vi "Update VI Properties.vi"() -> ()   [LabVIEW 2016, in "update vi properties.lvlib"]
uses:
  update vi properties.lvlib
  _support/user action.ctl
  _support/Event Data.ctl
  _support/Cluster_Data.ctl
  <vilib>/picture/picture.llb/imagedata.ctl
panel:
  in  "Add copyright":bool
  out "Inline?":bool
  out "Reentrant?":bool
  in  "Abbr. if class in lib":bool=TRUE
  in  "Adjust all Controls & Indicators":bool=TRUE
  in  "Prompt?":bool
  in  "Set all VIs":bool
  in  "Load":bool
  in  "Error in":errorcluster
  in  "Event Data":T1={"Action"=enum."Apply", "VI Index"=0}
  in  "Controls":string[][](table)
  in  "Indicators":string[][](table)
  in  "Help Tag":string
  in  "Help Path":string
  out "Path to VI":string
  in  "VI Description":string
  out "VI Conn Pane":picture
  in  "Listbox with VIs":i32(listbox)=-1 caption="Select a VI to View/Edit Properties:"
  in  "Action":T2=enum."Apply"
  in  "OK":bool
  in  "Cancel":bool
  in  "Apply":bool
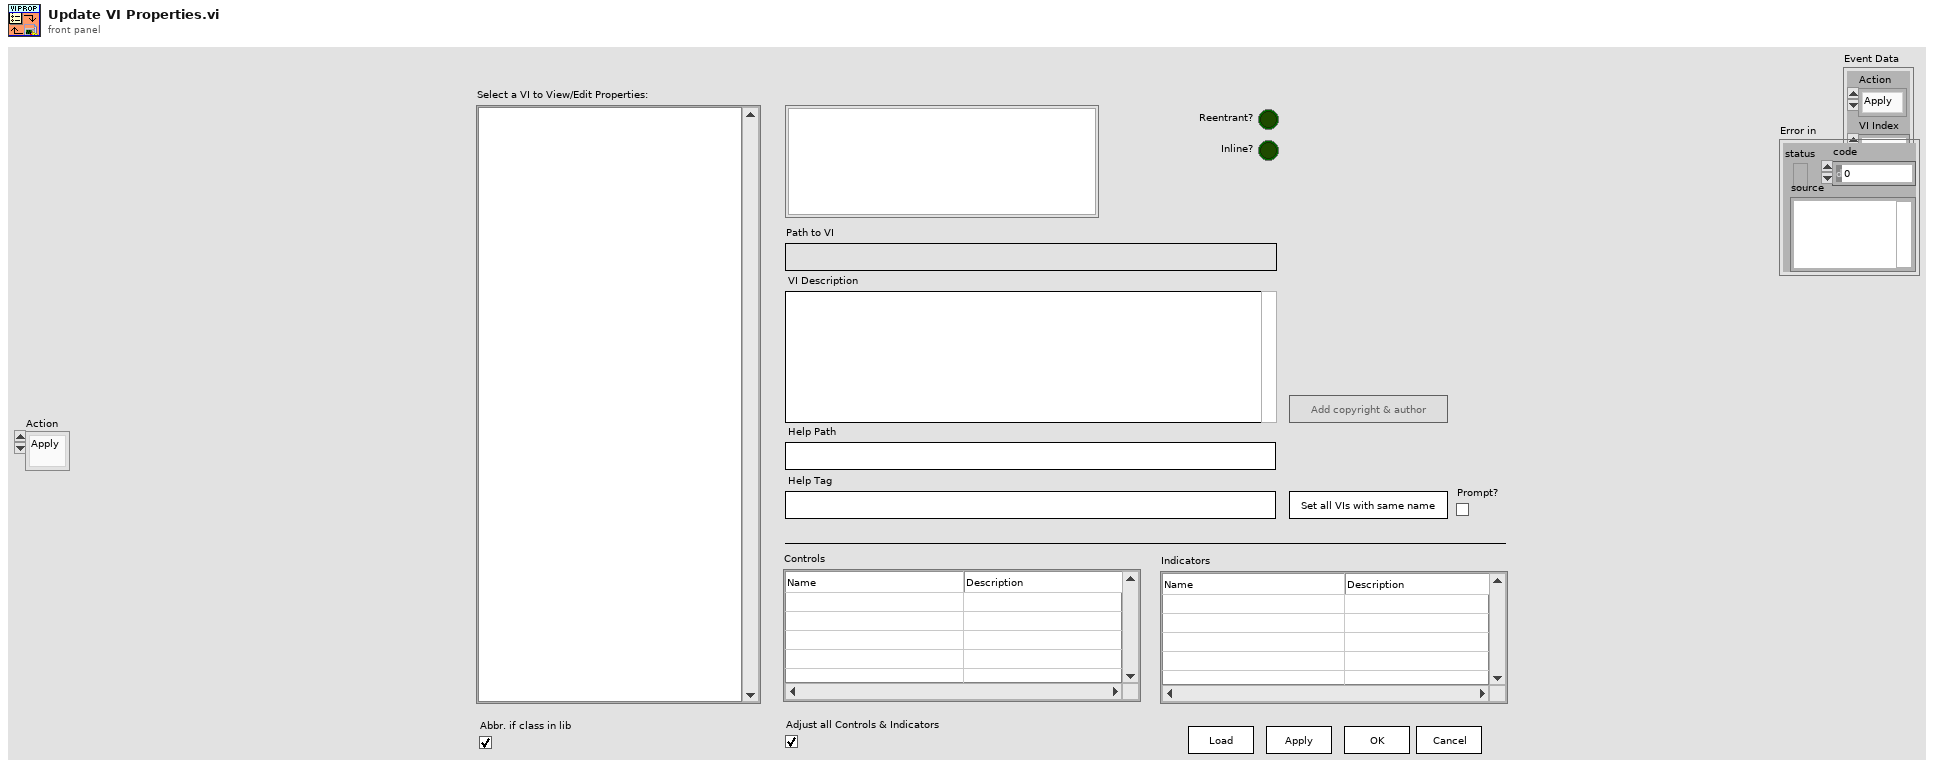
[diagram p1: front panel]
types:
  T1 = typedef "update vi properties.lvlib/Event Data.ctl" = cluster{"Action":T2, "VI Index":i32}
  T2 = typedef "update vi properties.lvlib/user action.ctl" = enum16{"Load VIs", "VI Selected", "Value Changed", "Set all VIs", "Controls/Indicator Changed", "Open VI", "Apply", "Cancel"}
  T3 = typedef "update vi properties.lvlib/Cluster_Data.ctl" = cluster{"changed?":bool, "VI Data":string[], "Controls":string[][], "Indicator":string[][], "Conpane Img":T4}
  T4 = typedef "imagedata.ctl" = cluster{"image type":i32, "image depth":i32, "image":u8[], "mask":u8[], "colors":u32[], "Rectangle":cluster{"left":i16, "top":i16, "right":i16, "bottom":i16}}
  T5 = enum32{"invalid VI type", "Standard VI", "Control VI", "Global VI", "Polymorphic VI", "Configuration VI", "SubSystem", "Facade VI", "Method VI", "Statechart Diagram VI"}
  T6 = enum8{"Enabled", "Disabled", "Disabled and Grayed Out"}
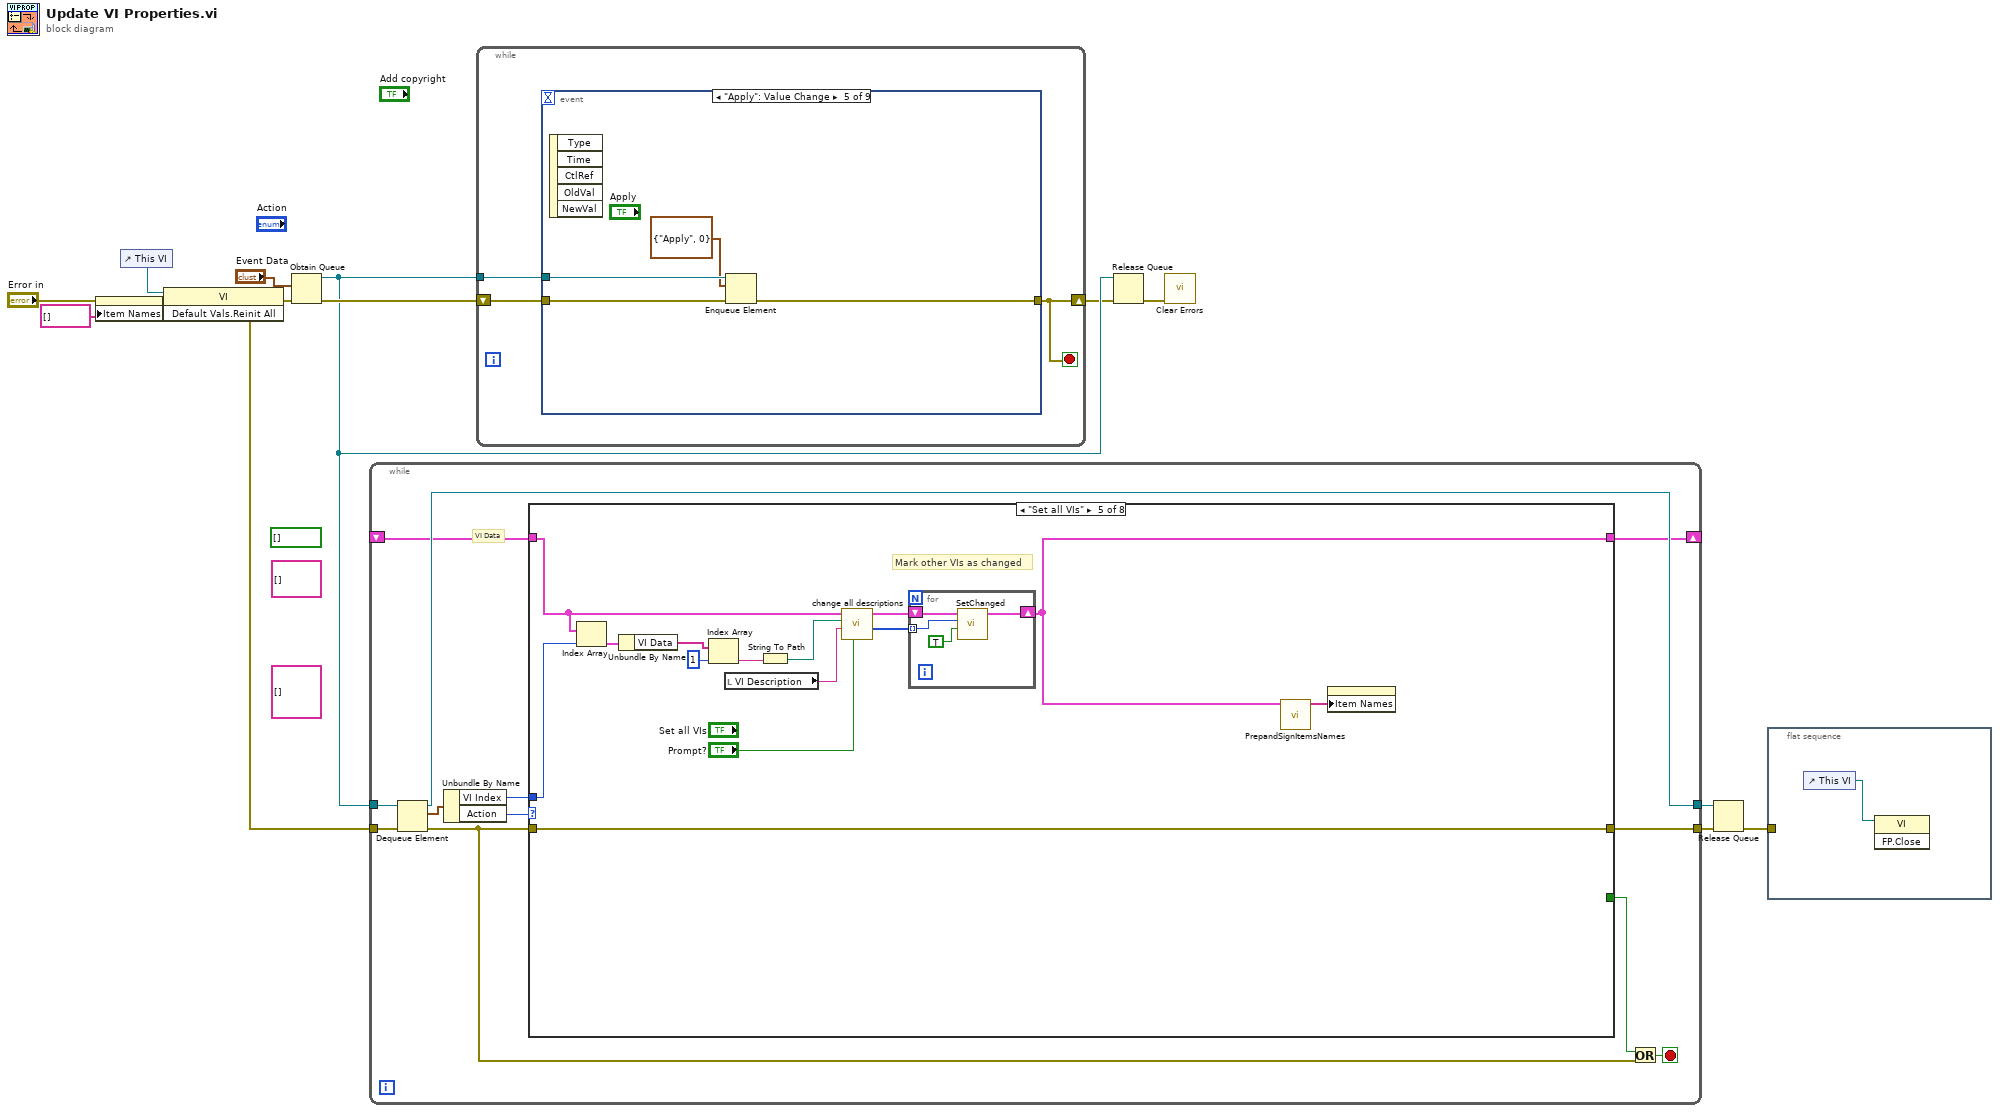
[diagram p0: block diagram]
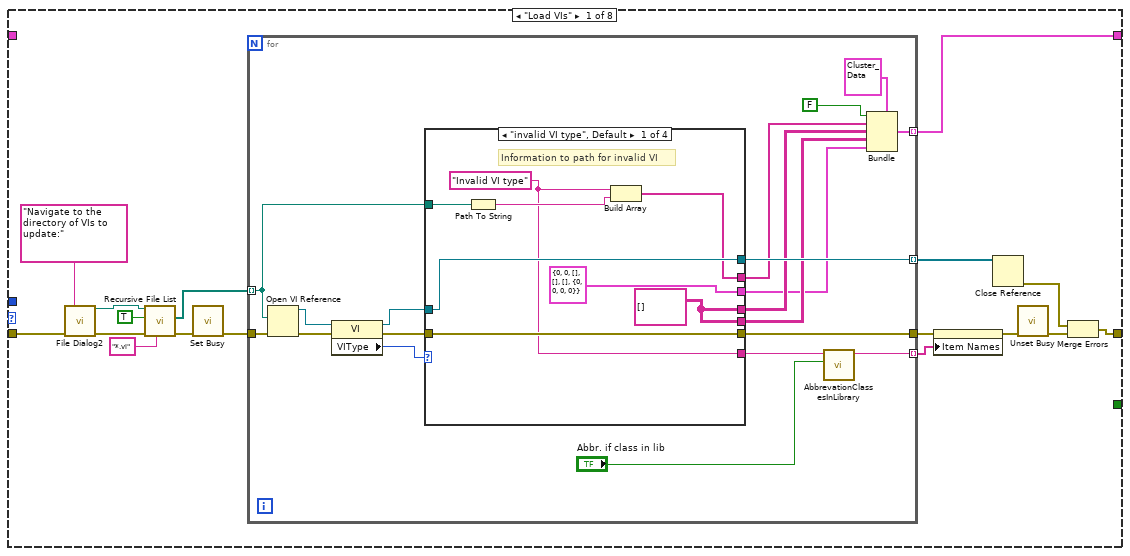
[diagram p2: hidden frame]
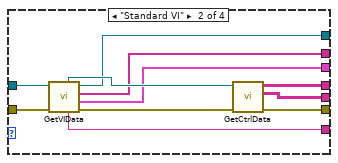
[diagram p3: hidden frame]
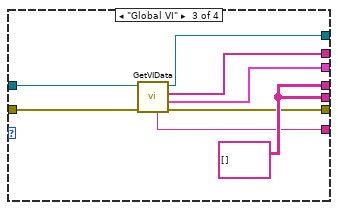
[diagram p4: hidden frame]
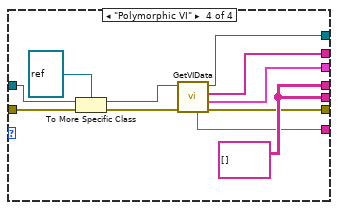
[diagram p5: hidden frame]
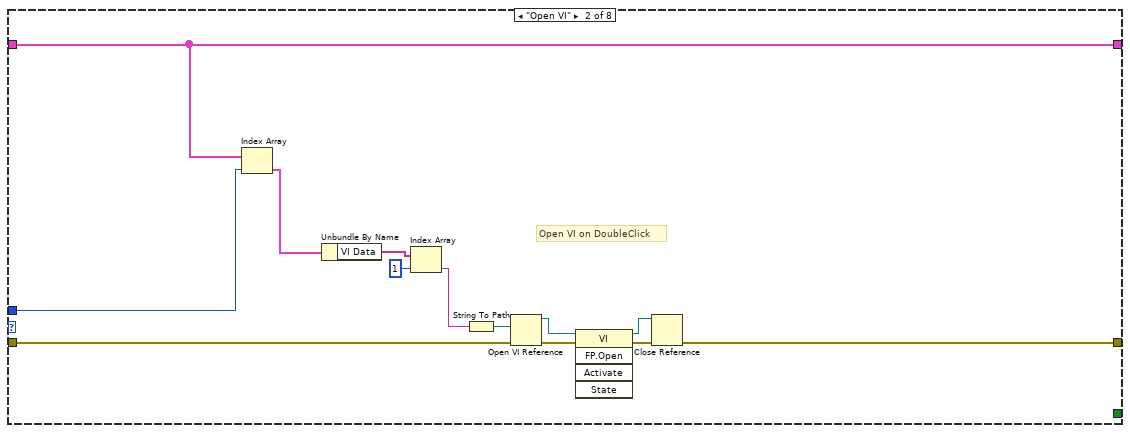
[diagram p6: hidden frame]
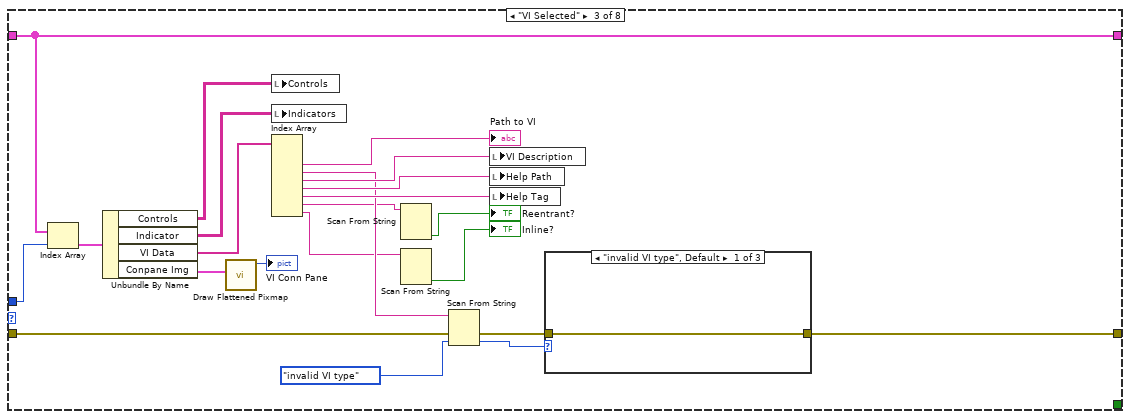
[diagram p7: hidden frame]
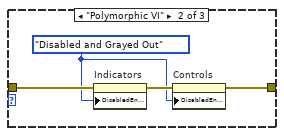
[diagram p8: hidden frame]
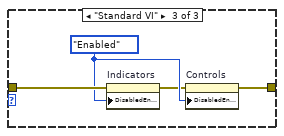
[diagram p9: hidden frame]
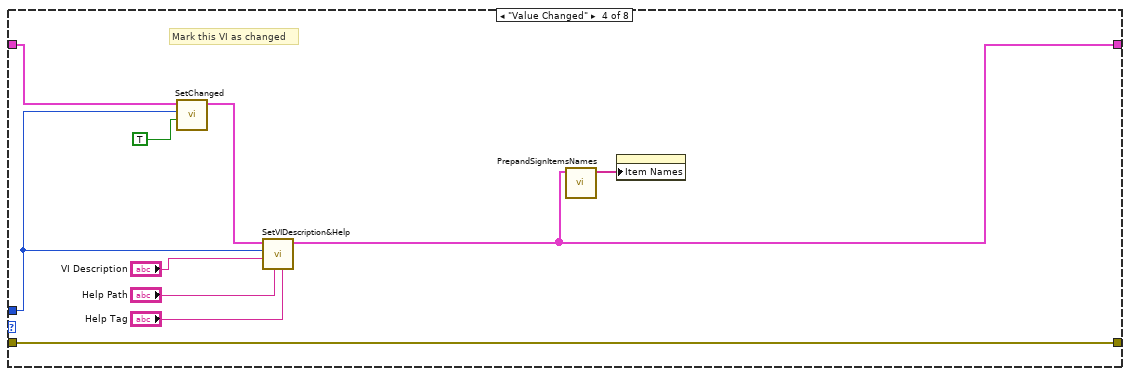
[diagram p10: hidden frame]
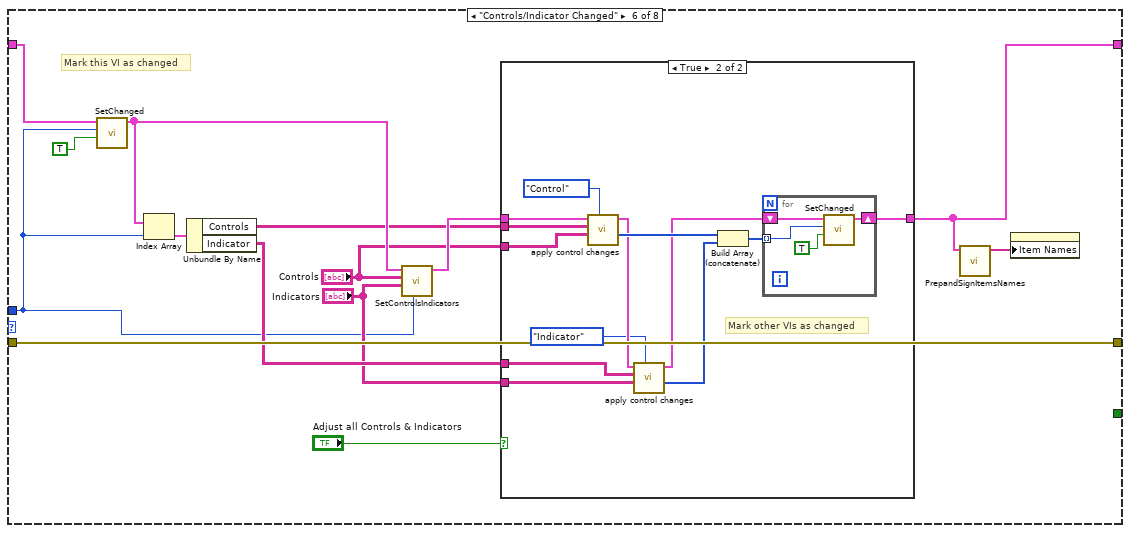
[diagram p11: hidden frame]
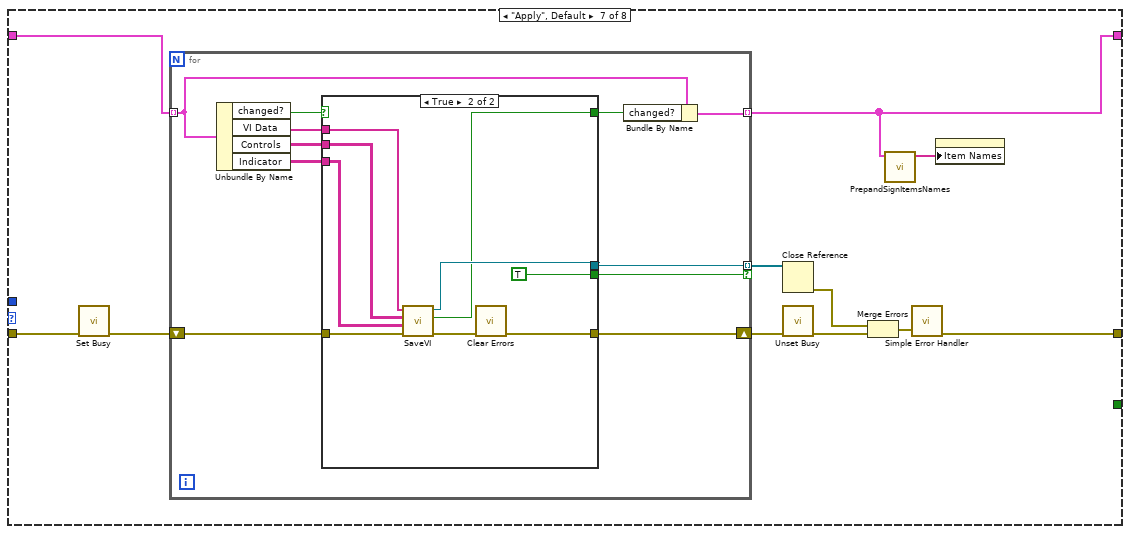
[diagram p13: hidden frame]
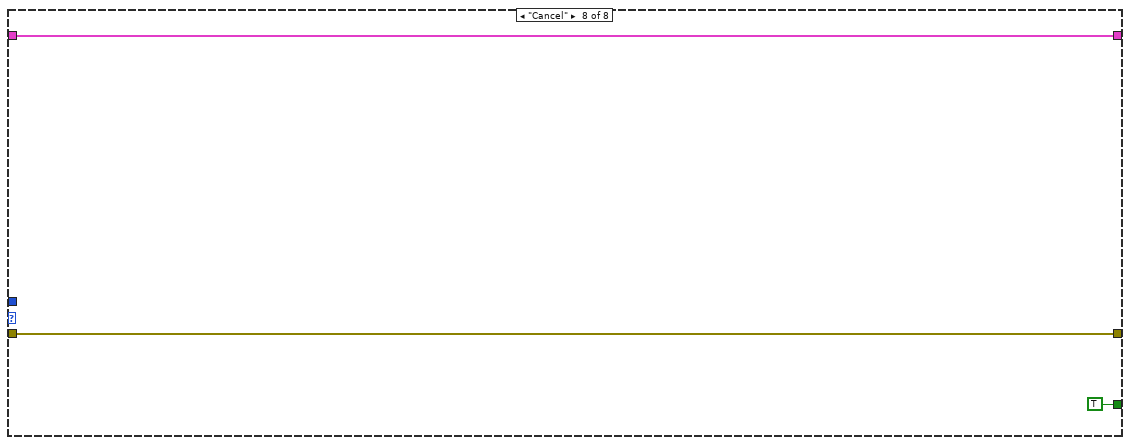
[diagram p15: hidden frame]
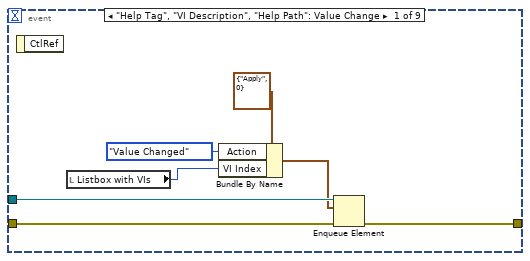
[diagram p16: hidden frame]
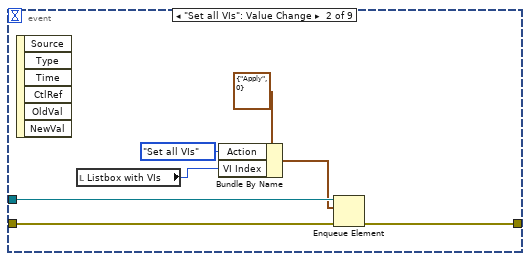
[diagram p17: hidden frame]
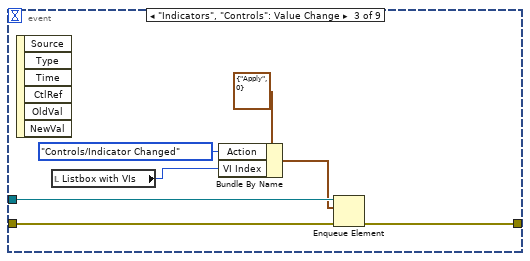
[diagram p18: hidden frame]
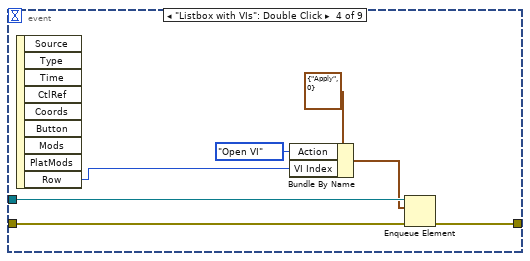
[diagram p19: hidden frame]
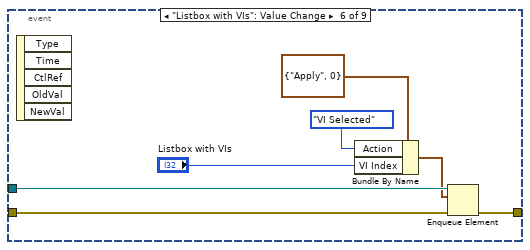
[diagram p20: hidden frame]
diagram:
  (unwired) string[][][] []
  (unwired) string[][] []
  (unwired) bool[] []
  n1 = property on="Listbox with VIs" class="LstBox (strict)"(error in="Error in", "Item Names"=string[] []) -> (error out=w5:errorcluster)  [unwired: 1 in, 1 out]
  n2 = control-ref of="This VI"() -> (w8:refnum<vi>)
  n3 = invoke class="VI" method="Default Vals.Reinit All"(reference=w8, error in=w5) -> (error out=w7:errorcluster)  [unwired: 1 in, 2 out]
  n4 = Obtain Queue(element data type="Event Data", error in (no error)=w7) -> (queue out=w9:refnum<queue>, error out=w10:errorcluster)  [unwired: 3 in, 1 out]
  n5 = while {
    tunnel: w7 -> [w21]
    tunnel: w9 -> [w25]
    tunnel: [w18] -> w13
    tunnel: [w24] -> w12
    shift-right: [w19] -> _
    shift-left: _ -> [w20]
    stop <- w15 stop-if-true
    # "VI Data"
    n6 = Dequeue Element(queue=w25, error in (no error)=w21) -> (queue out=w24:refnum<queue>, element=w23:T1, error out=w16:errorcluster)  [unwired: 1 in, 1 out]
    n7 = Unbundle By Name(w23) -> ("VI Index"=w22:i32, "Action"=w17:T2)
    n8 = case shown="\"Set all VIs\"" w17 {
      tunnel: w16 -> [w38 w107 w129 w153 w167 w185 w214 w240]
      tunnel: [_ _ _ _ _ _ _ TRUE] -> w14
      tunnel: [w27 w108 w126 w153 w167 w185 w207 w240] -> w18
      tunnel: w22 -> [_ w105 w128 w150 w156 w174 _ _]
      tunnel: w20 -> [_ w106 w125 w148 w164 w181 w206 w239]
      tunnel: [w26 w106 w125 w144 w155 w172 w204 w239] -> w19
      frame "Load VIs" {
        n9 = call "File Dialog2"("prompt"="Navigate to the directory of VIs to update:", "error in"=w38) -> ("selected path"=w40:path, "error out"=w41:errorcluster)  [unwired: 10 in, 2 out]
        n10 = call <vilib>:"Recursive File List.vi"("pattern"="*.vi", "error in (no error)"=w41, "Treat LLBs as Folders?"=TRUE, "Folder Path"=w40) -> ("error out"=w36:errorcluster, "All Files in Dir"=w34:path[])  [unwired: 3 in, 3 out]
        n11 = call <vilib>:"Set Busy.vi"("error in (no error)"=w36) -> ("error out"=w35:errorcluster)  [unwired: 9 in, 1 out]
        n12 = for {
          tunnel: w35 -> [w60]
          tunnel: w34 -> [w43] mode=indexing
          tunnel: [w46] -> w33 mode=indexing
          tunnel: [w56] -> w32
          tunnel: [w55] -> w30 mode=indexing
          tunnel: [w49] -> w26 mode=indexing
          n13 = Open VI Reference(vi path=w43, error in (no error)=w60) -> (vi reference=w44:refnum<vi>, error out=w61:errorcluster)  [unwired: 4 in]
          n14 = property class="VI"(reference=w44, error in=w61) -> (reference out=w58:refnum<vi>, error out=w59:errorcluster, "VIType"=w57:T5)
          n15 = case shown="\"invalid VI type\", Default" w57 {
            tunnel: w59 -> [w67 w80 w88 w98]
            tunnel: w58 -> [w66 w79 w82 w97]
            tunnel: [w65 w70 w84 w91] -> w54
            tunnel: [w62 w72 w85 w93] -> w45
            tunnel: [w69 w75 w87 w96] -> w53
            tunnel: [w69 w74 w87 w96] -> w52
            tunnel: [T4 {"image type"=0, "image depth"=0, "image"=[], "mask"=[], "colors"=[], "Rectangle"={"left"=0, "top"=0, "right"=0, "bottom"=0}} ("Get Conpane Image") w73 w83 w90] -> w51
            tunnel: [w67 w71 w86 w92] -> w56
            tunnel: [w66 w76 w81 w89] -> w55
            tunnel: w43 -> [w64 _ _ _]
            frame "invalid VI type", Default {
              w62 = "Invalid VI type" ("Help.Tag")
              w69 = string[][] []
              # "Information to path for invalid VI"
              n16 = Path To String(path=w64) -> (string=w63:string)
              n17 = Build Array(w62, w63) -> (w65:string[])
            }
            frame "Standard VI" {
              n18 = call "GetVIData.vi"("error in (no error)"=w80, "VI in"=w79) -> ("error out"=w78:errorcluster, "Get Conpane Image"=w73:T4, "Array"=w70:string[], "VI out"=w76:refnum<vi>, "Name"=w72:string, "Panel"=w77:refnum<vi>)  [unwired: 4 in]
              n19 = call "GetCtrlData.vi"("error in (no error)"=w78, "Panel in"=w77) -> ("error out"=w71:errorcluster, "Indicators"=w74:string[][], "Controls"=w75:string[][])  [unwired: 7 in]
            }
            frame "Global VI" {
              w87 = string[][] []
              n20 = call "GetVIData.vi"("error in (no error)"=w88, "VI in"=w82) -> ("error out"=w86:errorcluster, "Get Conpane Image"=w83:T4, "Array"=w84:string[], "VI out"=w81:refnum<vi>, "Name"=w85:string)  [unwired: 4 in, 1 out]
            }
            frame "Polymorphic VI" {
              w96 = string[][] []
              n21 = To More Specific Class(target class=refnum<vi> refnum, reference=w97, error in=w98) -> (specific class reference=w94:refnum<vi>, error out=w95:errorcluster)
              n22 = call "GetVIData.vi"("error in (no error)"=w95, "VI in"=w94) -> ("error out"=w92:errorcluster, "Get Conpane Image"=w90:T4, "Array"=w91:string[], "VI out"=w89:refnum<vi>, "Name"=w93:string)  [unwired: 4 in, 1 out]
            }
          }
          n23 = call "AbbrevationClassesInLibrary.vi"("Abbr. if class in lib"="Abbr. if class in lib", "Name in"=w45) -> ("Name out"=w46:string)  [unwired: 9 in]
          n24 = Bundle(cluster=T3 {"changed?"=FALSE, "VI Data"=[], "Controls"=[], "Indicator"=[], "Conpane Img"={"image type"=0, "image depth"=0, "image"=[], "mask"=[], "colors"=[], "Rectangle"={"left"=0, "top"=0, "right"=0, "bottom"=0}}}, "changed?"=FALSE, "VI Data"=w54, "Controls"=w53, "Indicator"=w52, "Conpane Img"=w51) -> (w49:T3)
        }
        n25 = property on="Listbox with VIs" class="LstBox (strict)"(error in=w32, "Item Names"=w33) -> (error out=w31:errorcluster)  [unwired: 1 in, 1 out]
        n26 = Close Reference(reference=w30) -> (error out=w29:errorcluster)  [unwired: 1 in]
        n27 = call <vilib>:"Unset Busy.vi"("error in (no error)"=w31) -> ("error out"=w28:errorcluster)  [unwired: 10 in]
        n28 = Merge Errors(w29, w28) -> (w27:errorcluster)
      }
      frame "Open VI" {
        # "Open VI on DoubleClick"
        n29 = Index Array(array=w106, index=w105) -> (element=w104:T3)
        n30 = Unbundle By Name(w104) -> ("VI Data"=w103:string[])
        n31 = Index Array(array=w103, index=1) -> (element=w102:string)
        n32 = String To Path(string=w102) -> (path=w101:path)
        n33 = Open VI Reference(vi path=w101, error in (no error)=w107) -> (vi reference=w111:refnum<vi>, error out=w112:errorcluster)  [unwired: 4 in]
        n34 = invoke class="VI" method="FP.Open"(reference=w111, error in=w112) -> (reference out=w109:refnum<vi>, error out=w110:errorcluster)  [unwired: 3 in, 3 out]
        n35 = Close Reference(reference=w109, error in (no error)=w110) -> (error out=w108:errorcluster)
      }
      frame "VI Selected" {
        n36 = Index Array(array=w125, index=w128) -> (element=w133:T3)
        n37 = Unbundle By Name(w133) -> ("Controls"=w121:string[][], "Indicator"=w122:string[][], "VI Data"=w123:string[], "Conpane Img"=w124:T4)
        n38 = call <vilib>:"Draw Flattened Pixmap.vi"("image data"=w124) -> ("new picture"=→"VI Conn Pane":picture)  [unwired: 8 in]
        n39 = local write "Controls"(w121) -> ()
        n40 = local write "Indicators"(w122) -> ()
        n41 = Index Array(array=w123) -> (element #2=→"Path to VI":string, element #3=w120:string, element #4=w132:string, element #5=w131:string, element #6=w130:string, element #7=w116:string, element #8=w114:string)  [unwired: 8 in, 1 out]
        n42 = Scan From String(input string=w116) -> (output 1=→"Reentrant?":bool)  [unwired: 4 in, 3 out]
        n43 = Scan From String(input string=w114) -> (output 1=→"Inline?":bool)  [unwired: 4 in, 3 out]
        n44 = Scan From String(input string=w120, error in=w129, default 1=T5."invalid VI type" ("VI Type")) -> (error out=w118:errorcluster, output 1=w117:T5)  [unwired: 2 in, 2 out]
        n45 = local write "VI Description"(w132) -> ()
        n46 = local write "Help Path"(w131) -> ()
        n47 = local write "Help Tag"(w130) -> ()
        n48 = case shown="\"invalid VI type\", Default" w117 {
          tunnel: w118 -> [w135 w138 w143]
          tunnel: [w135 w137 w140] -> w126
          frame "invalid VI type", Default {
          }
          frame "Polymorphic VI" {
            w136 = T6."Disabled and Grayed Out" ("Disabled")
            n49 = property on="Indicators" class="Tbl (strict)"(error in=w138, "DisabledEnum"=w136) -> (error out=w139:errorcluster)  [unwired: 1 in, 1 out]
            n50 = property on="Controls" class="Tbl (strict)"(error in=w139, "DisabledEnum"=w136) -> (error out=w137:errorcluster)  [unwired: 1 in, 1 out]
          }
          frame "Standard VI" {
            w142 = T6."Enabled" ("Disabled")
            n51 = property on="Indicators" class="Tbl (strict)"(error in=w143, "DisabledEnum"=w142) -> (error out=w141:errorcluster)  [unwired: 1 in, 1 out]
            n52 = property on="Controls" class="Tbl (strict)"(error in=w141, "DisabledEnum"=w142) -> (error out=w140:errorcluster)  [unwired: 1 in, 1 out]
          }
        }
      }
      frame "Value Changed" {
        # "Mark this VI as changed"
        n53 = call "SetChanged.vi"("changed?"=TRUE ("new element/subarray"), "VI Index"=w150, "Array in"=w148) -> ("Array out"=w147:T3[])  [unwired: 8 in]
        n54 = call "SetVIDescription&Help.vi"("Help Tag"="Help Tag", "Help Path"="Help Path", "VI Description"="VI Description", "VI Index"=w150, "VI Data in"=w147) -> ("VI Data out"=w144:T3[])  [unwired: 6 in]
        n55 = call "PrepandSignItemsNames.vi"("VI Data in"=w144) -> ("Array"=w145:string[])  [unwired: 10 in]
        n56 = property on="Listbox with VIs" class="LstBox (strict)"("Item Names"=w145) -> ()  [unwired: 2 in, 2 out]
      }
      frame "Set all VIs" {
        # "Mark other VIs as changed"
        n57 = Index Array(array=w164, index=w156) -> (element=w163:T3)
        n58 = Unbundle By Name(w163) -> ("VI Data"=w162:string[])
        n59 = Index Array(array=w162, index=1) -> (element=w160:string)
        n60 = local read "VI Description"() -> (w158:string)
        n61 = String To Path(string=w160) -> (path=w159:path)
        n62 = call "change all descriptions.vi"("Prompt?"="Prompt?", "new"=w158, "Path"=w159, "VI Data in"=w164) -> ("Changed indices"=w166:i32[], "VI Data out"=w165:T3[])  [unwired: 5 in, 1 out]
        n63 = for {
          shift-right: [w170] -> w155
          shift-left: w165 -> [w171]
          tunnel: w166 -> [w169] mode=indexing
          n64 = call "SetChanged.vi"("changed?"=TRUE ("new element/subarray"), "VI Index"=w169, "Array in"=w171) -> ("Array out"=w170:T3[])  [unwired: 8 in]
        }
        n65 = call "PrepandSignItemsNames.vi"("VI Data in"=w155) -> ("Array"=w154:string[])  [unwired: 10 in]
        n66 = property on="Listbox with VIs" class="LstBox (strict)"("Item Names"=w154) -> ()  [unwired: 2 in, 2 out]
      }
      frame "Controls/Indicator Changed" {
        # "Mark this VI as changed"
        n67 = call "SetChanged.vi"("changed?"=TRUE ("new element/subarray"), "VI Index"=w174, "Array in"=w181) -> ("Array out"=w178:T3[])  [unwired: 8 in]
        n68 = Index Array(array=w178, index=w174) -> (element=w184:T3)
        n69 = Unbundle By Name(w184) -> ("Controls"=w177:string[][], "Indicator"=w179:string[][])
        n70 = call "SetControlsIndicators.vi"("VI Index"=w174, "Indicators"="Indicators", "Controls"="Controls", "Data In"=w178) -> ("Data Out"=w183:T3[])  [unwired: 7 in]
        n71 = case shown="True" "Adjust all Controls & Indicators" {
          tunnel: "Controls" -> [_ w198]
          tunnel: w177 -> [_ w199]
          tunnel: w179 -> [_ w197]
          tunnel: "Indicators" -> [_ w196]
          tunnel: w183 -> [w186 w191]
          tunnel: [w186 w193] -> w172
          frame False {
          }
          frame True {
            # "Mark other VIs as changed"
            n72 = call "apply control changes.vi"("Type"=enum16{"Control", "Indicator"}."Control", "new"=w198, "old"=w199, "Data In"=w191) -> ("Changed indices"=w195:i32[], "Data Out"=w190:T3[])  [unwired: 6 in]
            n73 = call "apply control changes.vi"("Type"=enum16{"Control", "Indicator"}."Indicator", "new"=w196, "old"=w197, "Data In"=w190) -> ("Changed indices"=w194:i32[], "Data Out"=w189:T3[])  [unwired: 6 in]
            n74 = Build Array (concatenate)(w195, w194) -> (w192:i32[])
            n75 = for {
              shift-right: [w202] -> w193
              shift-left: w189 -> [w203]
              tunnel: w192 -> [w201] mode=indexing
              n76 = call "SetChanged.vi"("changed?"=TRUE ("new element/subarray"), "VI Index"=w201, "Array in"=w203) -> ("Array out"=w202:T3[])  [unwired: 8 in]
            }
          }
        }
        n77 = call "PrepandSignItemsNames.vi"("VI Data in"=w172) -> ("Array"=w173:string[])  [unwired: 10 in]
        n78 = property on="Listbox with VIs" class="LstBox (strict)"("Item Names"=w173) -> ()  [unwired: 2 in, 2 out]
      }
      frame "Apply", Default {
        n79 = call <vilib>:"Set Busy.vi"("error in (no error)"=w214) -> ("error out"=w213:errorcluster)  [unwired: 9 in, 1 out]
        n80 = for {
          shift-right: [w223] -> w212
          shift-left: w213 -> [w225]
          tunnel: w206 -> [w220] mode=indexing
          tunnel: [w224] -> w210 mode=indexing if=w222
          tunnel: [w218] -> w204 mode=indexing
          n81 = Unbundle By Name(w220) -> ("changed?"=w221:bool, "VI Data"=w217:string[], "Controls"=w216:string[][], "Indicator"=w215:string[][])
          n82 = case shown="True" w221 {
            selector: w221 -> [w226 _]
            tunnel: w217 -> [_ w238]
            tunnel: w225 -> [w228 w237]
            tunnel: [refnum<k0> refnum w236] -> w224
            tunnel: [w228 w235] -> w223
            tunnel: [FALSE TRUE] -> w222
            tunnel: [w226 w232] -> w219
            tunnel: w216 -> [_ w231]
            tunnel: w215 -> [_ w230]
            frame False {
            }
            frame True {
              n83 = call "SaveVI.vi"("error in (no error)"=w237, "Indicator"=w230, "Controls"=w231, "Data"=w238) -> ("error out"=w233:errorcluster, "status"=w232:bool, "VI out"=w236:refnum<vi>)  [unwired: 5 in]
              n84 = call <vilib>:"Clear Errors.vi"("error in (no error)"=w233) -> ("error out"=w235:errorcluster)  [unwired: 5 in, 1 out]
            }
          }
          n85 = Bundle By Name(cluster=w220, "changed?"=w219) -> (w218:T3)
        }
        n86 = Close Reference(reference=w210) -> (error out=w208:errorcluster)  [unwired: 1 in]
        n87 = call <vilib>:"Unset Busy.vi"("error in (no error)"=w212) -> ("error out"=w211:errorcluster)  [unwired: 10 in]
        n88 = Merge Errors(w208, w211) -> (w209:errorcluster)
        n89 = call "PrepandSignItemsNames.vi"("VI Data in"=w204) -> ("Array"=w205:string[])  [unwired: 10 in]
        n90 = call <vilib>:"Simple Error Handler.vi"("error in (no error)"=w209) -> ("error out"=w207:errorcluster)  [unwired: 4 in, 4 out]
        n91 = property on="Listbox with VIs" class="LstBox (strict)"("Item Names"=w205) -> ()  [unwired: 2 in, 2 out]
      }
      frame "Cancel" {
      }
    }
    n92 = Or(x=w14, y=w16) -> (x .or. y?=w15:bool)
  }
  n93 = while {
    shift-right: [w242] -> w3
    shift-left: w10 -> [w243]
    tunnel: w9 -> [w244]
    stop <- w242 stop-if-true
    n94 = event shown="[4] \"Apply\": Value Change" {
      selector: _ -> [_ _ _ _ _ _ _ _ _]
      dyn-events: _ -> [_ _ _ _ _ _ _ _ _]
      timeout: _ -> [_ _ _ _ _ _ _ _ _]
      tunnel: w244 -> [w251 w258 w265 w272 w276 w283 w287 w293 w297]
      tunnel: w243 -> [w250 w257 w264 w271 w275 w282 w286 w294 w296]
      tunnel: [w249 w256 w263 w270 w274 w278 errorcluster {"status"=TRUE, "code"=0, "source"=""} ("error out") w290 w295] -> w242
      event "Help Tag", "VI Description", "Help Path": Value Change {
        n95 = event-data() -> ()  [unwired: 1 in, 1 out]
        n96 = local read "Listbox with VIs"() -> (w246:i32)
        n97 = Bundle By Name(cluster=T1 {"Action"=enum."Apply", "VI Index"=0} ("element"), "Action"=user_action."Value Changed", "VI Index"=w246) -> (w245:T1)
        n98 = Enqueue Element(queue=w251, element=w245, error in (no error)=w250) -> (error out=w249:errorcluster)  [unwired: 1 in, 2 out]
      }
      event "Set all VIs": Value Change {
        n99 = event-data() -> ()  [unwired: 1 in, 6 out]
        n100 = local read "Listbox with VIs"() -> (w253:i32)
        n101 = Bundle By Name(cluster=T1 {"Action"=enum."Apply", "VI Index"=0} ("element"), "Action"=user_action."Set all VIs", "VI Index"=w253) -> (w252:T1)
        n102 = Enqueue Element(queue=w258, element=w252, error in (no error)=w257) -> (error out=w256:errorcluster)  [unwired: 1 in, 2 out]
      }
      event "Indicators", "Controls": Value Change {
        n103 = event-data() -> ()  [unwired: 1 in, 6 out]
        n104 = local read "Listbox with VIs"() -> (w260:i32)
        n105 = Bundle By Name(cluster=T1 {"Action"=enum."Apply", "VI Index"=0} ("element"), "Action"=user_action."Controls/Indicator Changed", "VI Index"=w260) -> (w259:T1)
        n106 = Enqueue Element(queue=w265, element=w259, error in (no error)=w264) -> (error out=w263:errorcluster)  [unwired: 1 in, 2 out]
      }
      event "Listbox with VIs": Double Click {
        n107 = event-data() -> ("Row"=w266:i32)  [unwired: 1 in, 8 out]
        n108 = Bundle By Name(cluster=T1 {"Action"=enum."Apply", "VI Index"=0} ("element"), "Action"=user_action."Open VI", "VI Index"=w266) -> (w267:T1)
        n109 = Enqueue Element(queue=w272, element=w267, error in (no error)=w271) -> (error out=w270:errorcluster)  [unwired: 1 in, 2 out]
      }
      event "Apply": Value Change {
        n110 = event-data() -> ()  [unwired: 1 in, 5 out]
        n111 = Enqueue Element(queue=w276, element=T1 {"Action"=enum."Apply", "VI Index"=0}, error in (no error)=w275) -> (error out=w274:errorcluster)  [unwired: 1 in, 2 out]
      }
      event "Listbox with VIs": Value Change {
        n112 = event-data() -> ()  [unwired: 1 in, 5 out]
        n113 = Bundle By Name(cluster=T1 {"Action"=enum."Apply", "VI Index"=0} ("element"), "Action"=user_action."VI Selected", "VI Index"="Listbox with VIs") -> (w279:T1)
        n114 = Enqueue Element(queue=w283, element=w279, error in (no error)=w282) -> (error out=w278:errorcluster)  [unwired: 1 in, 2 out]
      }
      event "Cancel": Value Change {
        # "True to Exit"
        n115 = event-data() -> ()  [unwired: 1 in, 5 out]
        n116 = Enqueue Element(queue=w287, element=T1 {"Action"=enum."Cancel", "VI Index"=0}, error in (no error)=w286) -> ()  [unwired: 1 in, 3 out]
      }
      event "OK": Value Change {
        n117 = event-data() -> ()  [unwired: 1 in, 5 out]
        n118 = Enqueue Element(queue=w293, element=T1 {"Action"=enum."Apply", "VI Index"=0}, error in (no error)=w294) -> (queue out=w291:refnum<queue>, error out=w292:errorcluster)  [unwired: 1 in, 1 out]
        n119 = Enqueue Element(queue=w291, element=T1 {"Action"=enum."Cancel", "VI Index"=0}, error in (no error)=w292) -> (error out=w290:errorcluster)  [unwired: 1 in, 2 out]
      }
      event "Load": Value Change {
        n120 = event-data() -> ()  [unwired: 1 in, 5 out]
        n121 = Enqueue Element(queue=w297, element=T1 {"Action"=enum."Load VIs", "VI Index"=0}, error in (no error)=w296) -> (error out=w295:errorcluster)  [unwired: 1 in, 2 out]
      }
    }
  }
  n122 = Release Queue(queue=w9, error in (no error)=w3) -> (error out=w1:errorcluster)  [unwired: 1 in, 2 out]
  n123 = call <vilib>:"Clear Errors.vi"("error in (no error)"=w1) -> ()  [unwired: 5 in, 2 out]
  n124 = Release Queue(queue=w12, error in (no error)=w13) -> (error out=w2:errorcluster)  [unwired: 1 in, 2 out]
  n125 = flat-sequence {
    tunnel: w2 -> [_]
    frame #0 {
      n126 = control-ref of="This VI"() -> (w299:refnum<vi>)
      n127 = invoke class="VI" method="FP.Close"(reference=w299) -> ()  [unwired: 2 in, 3 out]
    }
  }
